vi "case-structure1.vi"() -> ()   [LabVIEW 2025]
panel:
  out "result":i32
  in  "b":i32
  in  "a":i32
  in  "Boolean":bool
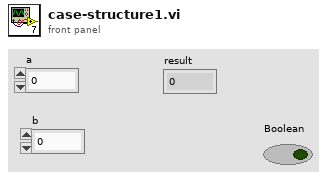
[diagram p1: front panel]
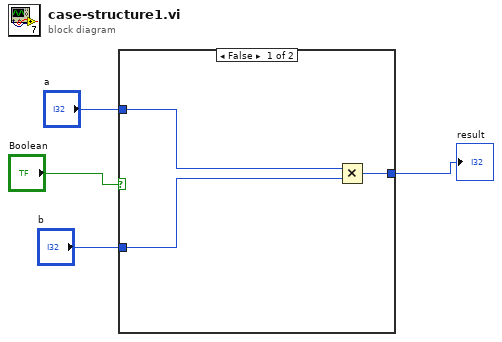
[diagram p0: block diagram]
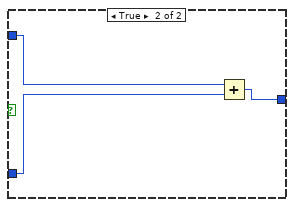
[diagram p2: hidden frame]
diagram:
  n1 = case shown="False" "Boolean" {
    tunnel: "a" -> [w7 w10]
    tunnel: "b" -> [w6 w9]
    tunnel: [w5 w8] -> w1
    frame False {
      n2 = Multiply(x=w7, y=w6) -> (x*y=w5:i32)
    }
    frame True {
      n3 = Add(x=w10, y=w9) -> (x+y=w8:i32)
    }
  }
  "result" <- w1
